vi "writeU8.vi"(8 "error in (no error)":errorcluster, 10 "Input":u8, 11 "M1M3SAL in":refnum<class "M1M3SAL.lvclass">) -> (0 "error out":errorcluster, 3 "M1M3SAL out":refnum<class "M1M3SAL.lvclass">)   [LabVIEW 2016, in "M1M3SupportCommunicator.lvlib" / "M1M3SAL.lvclass"]
uses:
  M1M3SAL.lvclass
  M1M3SAL.lvclass/M1M3SAL.ctl
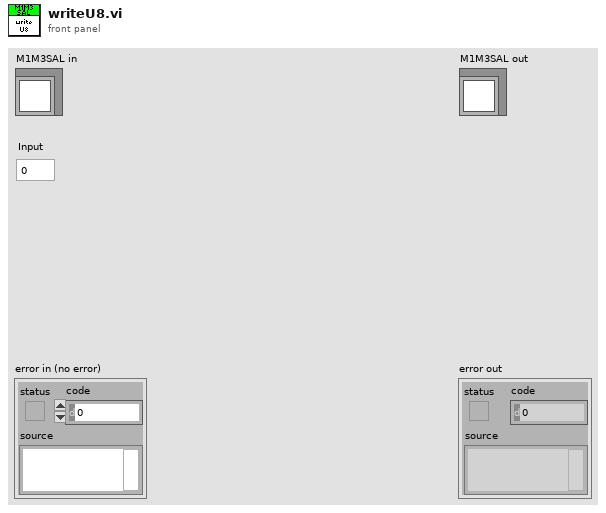
[diagram p1: front panel]
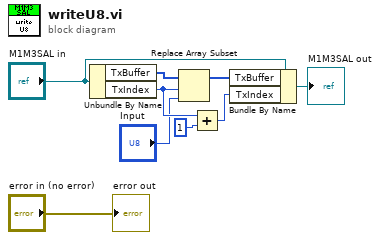
[diagram p0: block diagram]
diagram:
  n1 = Unbundle By Name("M1M3SAL in") -> ("TxBuffer"=w7:u8[], "TxIndex"=w6:i32)
  n2 = Replace Array Subset(array=w7, new element="Input", index=w6) -> (w2:u8[])
  n3 = Add(x=w6, y=1) -> (x+y=w4:i32)
  n4 = Bundle By Name(cluster="M1M3SAL in", "TxBuffer"=w2, "TxIndex"=w4) -> (→"M1M3SAL out":refnum<class "M1M3SAL.lvclass">)
  "error out" <- "error in (no error)"
